vi "Init Msg.vi"(6 "Teller":refnum<class "Teller.lvclass">) -> (2 "Msg":refnum<class "Msg.lvclass">)   [LabVIEW 2020, in "jettl.lvlib" / "Stopping jettl Msg.lvlib" / "Stopping.lvlib"]
doc: "jettl 6.12.1.94\nNathan Davis - Nathan Davis\nCopyright (c) 2026, Nathan Davis\nMIT"
uses:
  Stopping.lvlib
  Msg/Msg.lvclass
  Teller/Teller.lvclass
  Stopping Msg Input/Stopping Msg Input.lvlib
  Stopping Msg/Stopping Msg.lvlib
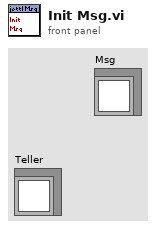
[diagram p1: front panel]
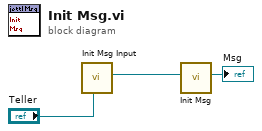
[diagram p0: block diagram]
diagram:
  n1 = call "Init Msg Input.vi"("Teller"="Teller") -> ("Msg Input"=w3:refnum<class "Msg Input.lvclass">)  [unwired: 10 in]
  n2 = call "Init Msg.vi"("Msg Input"=w3) -> ("Msg"=→"Msg":refnum<class "Msg.lvclass">)  [unwired: 10 in]
